vi "Read File Refnum.vi"(8 "error in (no error)":errorcluster, 11 "read file in":refnum<class "Read File.lvclass">) -> (0 "error out":errorcluster, 2 "file refnum":refnum<file>, 3 "read file out":refnum<class "Read File.lvclass">)   [LabVIEW 2023, in "read file.lvclass"]
doc: "Gets the file reference number from Read File.ctl."
uses:
  Read File.lvclass
  Read File.lvclass/Read File.ctl
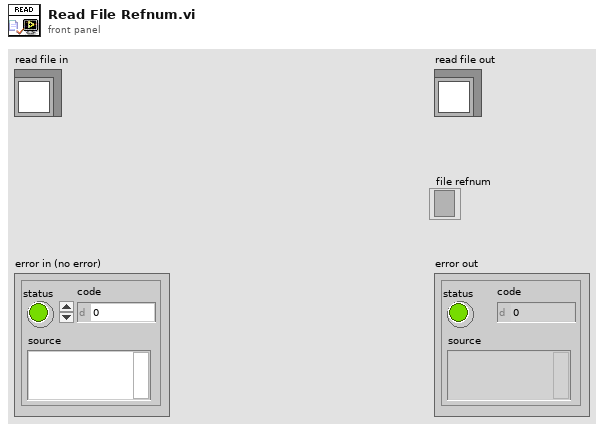
[diagram p1: front panel]
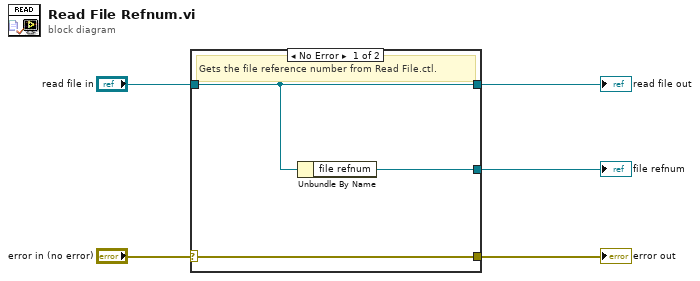
[diagram p0: block diagram]
diagram:
  n1 = case shown="No Error" "error in (no error)" {
    selector: "error in (no error)" -> [w8 w9]
    tunnel: [w8 w9] -> w4
    tunnel: [w7 w10] -> w2
    tunnel: "read file in" -> [w7 w10]
    tunnel: [w6 _] -> w1
    frame No Error {
      # "Gets the file reference number from Read File.ctl."
      n2 = Unbundle By Name(w7) -> ("file refnum"=w6:refnum<file>)
    }
    frame Error {
    }
  }
  "error out" <- w4
  "read file out" <- w2
  "file refnum" <- w1
